vi "OpenAny.vi"(8 "error in":errorcluster) -> (0 "error out":errorcluster, 1 "Address Found":string, 2 "Device Type Found":string, 3 "Handle":i32)   [LabVIEW 2021]
panel:
  # "None\nLJ_dtU3\nLJ_dtU6\nLJ_dtUE9"
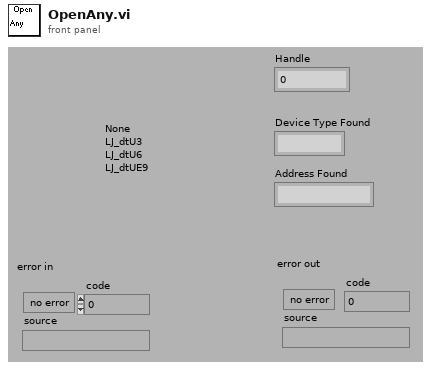
[diagram p1: front panel]
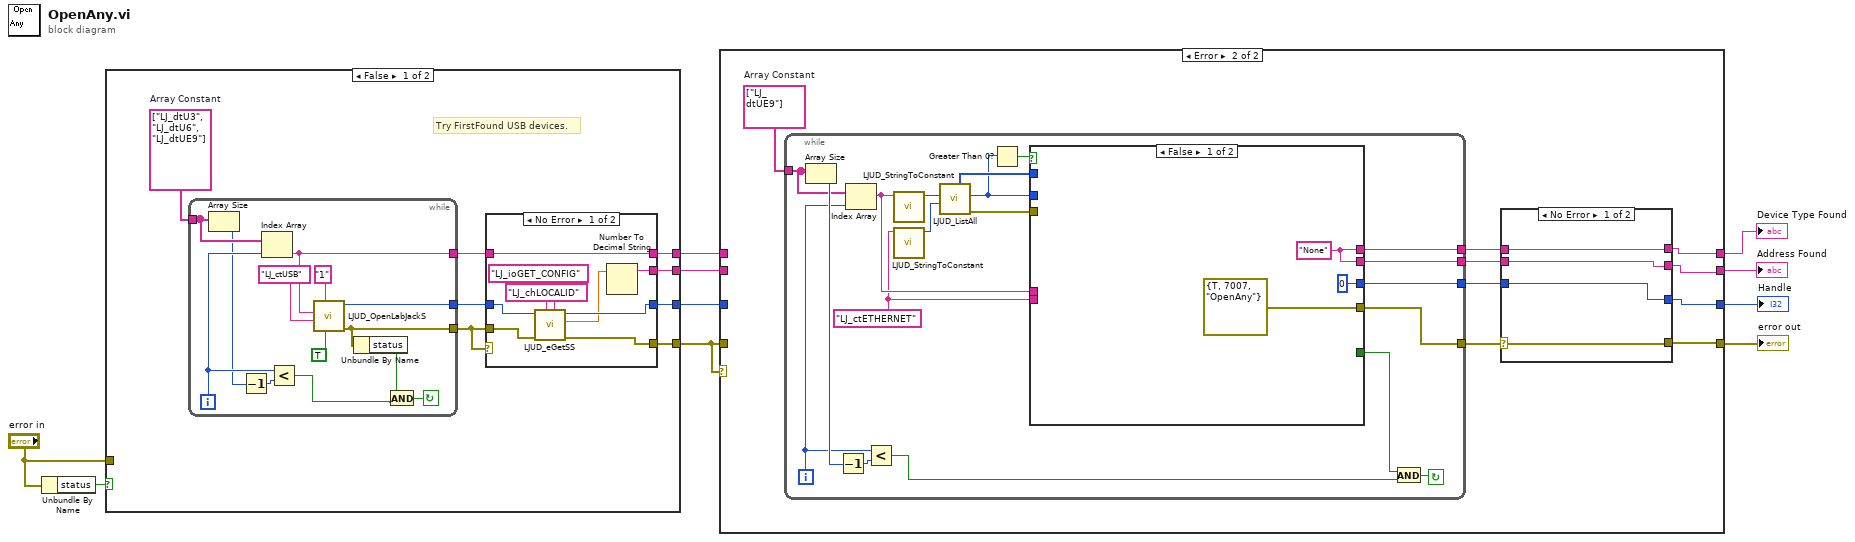
[diagram p0: block diagram]
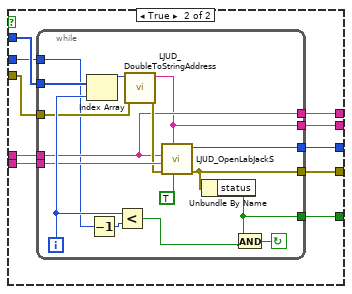
[diagram p3: hidden frame]
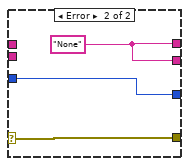
[diagram p4: hidden frame]
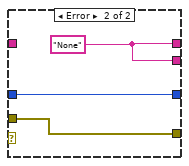
[diagram p5: hidden frame]
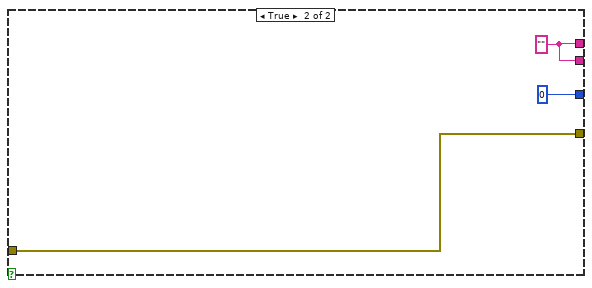
[diagram p6: hidden frame]
diagram:
  n1 = Unbundle By Name("error in") -> ("status"=w10:bool)
  n2 = case shown="False" w10 {
    tunnel: [w16 w44] -> w4
    tunnel: [w12 0 ("Handle")] -> w6
    tunnel: [w13 w46] -> w8
    tunnel: "error in" -> [_ w46]
    tunnel: [w11 w44] -> w2
    frame False {
      w17 = string[] ["LJ_dtU3", "LJ_dtU6", "LJ_dtUE9"]  # Array Constant
      # "Try FirstFound USB devices."
      n3 = while {
        tunnel: [w27] -> w18
        tunnel: w17 -> [w24]
        tunnel: [w25] -> w14
        tunnel: [w28] -> w15
        i -> [w23]
        stop <- w26 continue-if-true
        n4 = Array Size(array=w24) -> (size(s)=w21:i32)
        n5 = Decrement(x=w21) -> (x-1=w22:i32)
        n6 = Index Array(array=w24, index=w23) -> (element=w27:string)
        n7 = Less?(x=w23, y=w22) -> (x < y?=w19:bool)
        n8 = call "LJUD_OpenLabJackS.vi"("FirstFound"=TRUE, "Address"="1", "ConnectionType"="LJ_ctUSB", "DeviceType"=w27) -> ("error out"=w25:errorcluster, "Handle"=w28:i32)  [unwired: 5 in, 1 out]
        n9 = Unbundle By Name(w25) -> ("status"=w20:bool)
        n10 = And(x=w20, y=w19) -> (x .and. y?=w26:bool)
      }
      n11 = case shown="No Error" w14 {
        tunnel: w18 -> [w40 _]
        tunnel: [w40 w41] -> w16
        tunnel: w15 -> [w37 w42]
        tunnel: w14 -> [w36 w43]
        tunnel: [w35 w43] -> w13
        tunnel: [w34 w42] -> w12
        tunnel: [w32 w41] -> w11
        frame No Error {
          n12 = call "LJUD_eGetSS.vi"("Channel"="LJ_chLOCALID", "IOType"="LJ_ioGET_CONFIG", "error in"=w36, "Handle In"=w37) -> ("error out"=w35:errorcluster, "Value Read"=w33:dbl, "Handle Out"=w34:i32)  [unwired: 5 in]
          n13 = Number To Decimal String(number=w33) -> (decimal integer string=w32:string)  [unwired: 1 in]
        }
        frame Error {
          w41 = "None"
        }
      }
    }
    frame True {
      w44 = ""
    }
  }
  n14 = case shown="Error" w8 {
    tunnel: w8 -> [w50 _]
    tunnel: [w50 w51] -> w7
    tunnel: w6 -> [w49 _]
    tunnel: [w49 w53] -> w5
    tunnel: w4 -> [w48 _]
    tunnel: [w48 w57] -> w3
    tunnel: w2 -> [w47 _]
    tunnel: [w47 w55] -> w1
    frame No Error {
    }
    frame Error {
      w59 = string[] ["LJ_dtUE9"]  # Array Constant
      n15 = while {
        tunnel: [w62] -> w54
        tunnel: [w63] -> w56
        tunnel: [w64] -> w58
        tunnel: [w65] -> w52
        tunnel: w59 -> [w76]
        i -> [w75]
        stop <- w69 continue-if-true
        w67 = "LJ_ctETHERNET" ("ConnectionType")
        n16 = Array Size(array=w76) -> (size(s)=w77:i32)
        n17 = Decrement(x=w77) -> (x-1=w78:i32)
        n18 = Index Array(array=w76, index=w75) -> (element=w71:string)
        n19 = Less?(x=w75, y=w78) -> (x < y?=w70:bool)
        n20 = call "LJUD_StringToConstant.vi"("String"=w71) -> ("Constant Number"=w74:i32)  [unwired: 9 in, 1 out]
        n21 = call "LJUD_StringToConstant.vi"("String"=w67) -> ("Constant Number"=w73:i32)  [unwired: 9 in, 1 out]
        n22 = call "LJUD_ListAll.vi"("ConnectionType"=w73, "DeviceType"=w74) -> ("error out"=w61:errorcluster, "NumFound"=w60:i32, "Addresses"=w68:i32[])  [unwired: 5 in, 2 out]
        n23 = Greater Than 0?(x=w60) -> (x > 0?=w72:bool)
        n24 = case shown="False" w72 {
          tunnel: w71 -> [_ w92]
          tunnel: w68 -> [_ w91]
          tunnel: w67 -> [_ w90]
          tunnel: [TRUE ("status") w89] -> w66
          tunnel: [errorcluster {"status"=TRUE, "code"=7007, "source"="OpenAny"} ("error out") w88] -> w65
          tunnel: [w81 w87] -> w64
          tunnel: [w81 w86] -> w63
          tunnel: [0 ("Handle") w85] -> w62
          tunnel: w61 -> [_ w84]
          tunnel: w60 -> [_ w83]
          frame False {
            w81 = "None"
          }
          frame True {
            n25 = while {
              tunnel: w84 -> [w94]
              tunnel: [w95] -> w86
              tunnel: [w96] -> w87
              tunnel: [w97] -> w89
              tunnel: w90 -> [w99]
              tunnel: w92 -> [w96]
              tunnel: w91 -> [w104]
              tunnel: [w105] -> w88
              tunnel: [w107] -> w85
              tunnel: w83 -> [w93]
              i -> [w103]
              stop <- w106 continue-if-true
              n26 = Index Array(array=w104, index=w103) -> (element=w100:i32)
              n27 = Decrement(x=w93) -> (x-1=w102:i32)
              n28 = Less?(x=w103, y=w102) -> (x < y?=w101:bool)
              n29 = call "LJUD_DoubleToStringAddress.vi"("error in"=w94, "Double"=w100) -> ("error out"=w98:errorcluster, "String"=w95:string)  [unwired: 8 in]
              n30 = call "LJUD_OpenLabJackS.vi"("FirstFound"=TRUE, "Address"=w95, "error in"=w98, "ConnectionType"=w99, "DeviceType"=w96) -> ("error out"=w105:errorcluster, "Handle"=w107:i32)  [unwired: 4 in, 1 out]
              n31 = Unbundle By Name(w105) -> ("status"=w97:bool)
              n32 = And(x=w97, y=w101) -> (x .and. y?=w106:bool)
            }
          }
        }
        n33 = And(x=w66, y=w70) -> (x .and. y?=w69:bool)
      }
      n34 = case shown="No Error" w52 {
        selector: w52 -> [w109 w114]
        tunnel: [w112 w115] -> w57
        tunnel: [w109 w114] -> w51
        tunnel: [w110 w113] -> w53
        tunnel: [w111 w115] -> w55
        tunnel: w58 -> [w112 _]
        tunnel: w56 -> [w111 _]
        tunnel: w54 -> [w110 w113]
        frame No Error {
        }
        frame Error {
          w115 = "None"
        }
      }
    }
  }
  "error out" <- w7
  "Handle" <- w5
  "Device Type Found" <- w3
  "Address Found" <- w1
